vi "barcodeR092B.vi"(8 "主码":string, 10 "固定码":cluster{"start row":i32, "start column":i32}={"start row"=2, "start column"=1}) -> (2 "R92A二维码":string)   [LabVIEW 2020]
uses:
  Sources/Global_Variable/Global.vi
panel:
  out "结果字符串":string
  out "校验码":string="4"
  out "校验码数组":string[](array[string])=["0", "1", "2", "3", "4", "5", "6", "7", "8", "9", "A", "B", "C", "D", "E", "F", "G", "H", "J", "K", "L", "M", "N", "P", "R", "S", "T", "U", "V", "W", "X", "Y", "Z"]
  out "月份字码对照月校验数组":string[](array[string])=["", "", "", "", "", "", "", "", "", "", "01", "02", "03", "04", "05", "06", "07", "08", "09", "10", "11", "12"]
  out "批次流水号码":string
  out "年月日":string
  out "年月日时分码":string
  out "日期/时间字符串":string
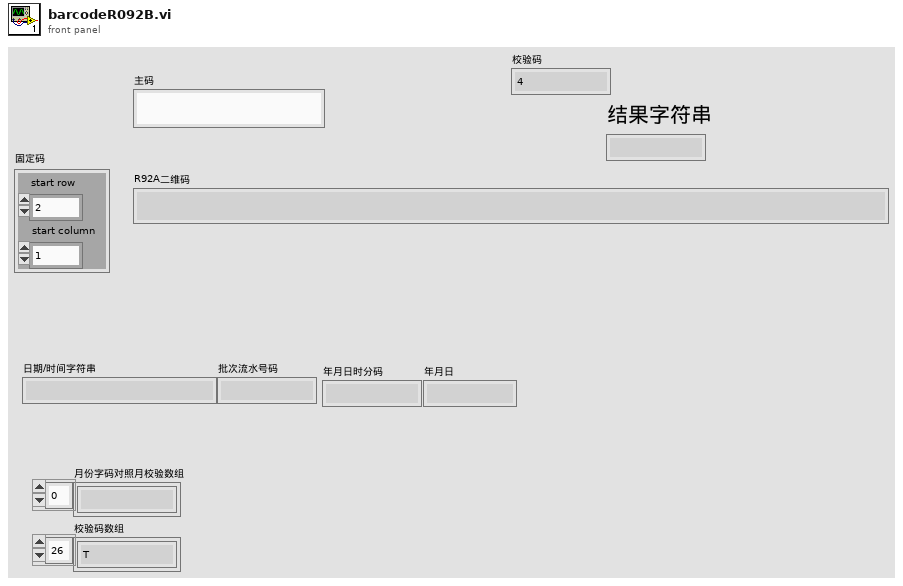
[diagram p1: front panel]
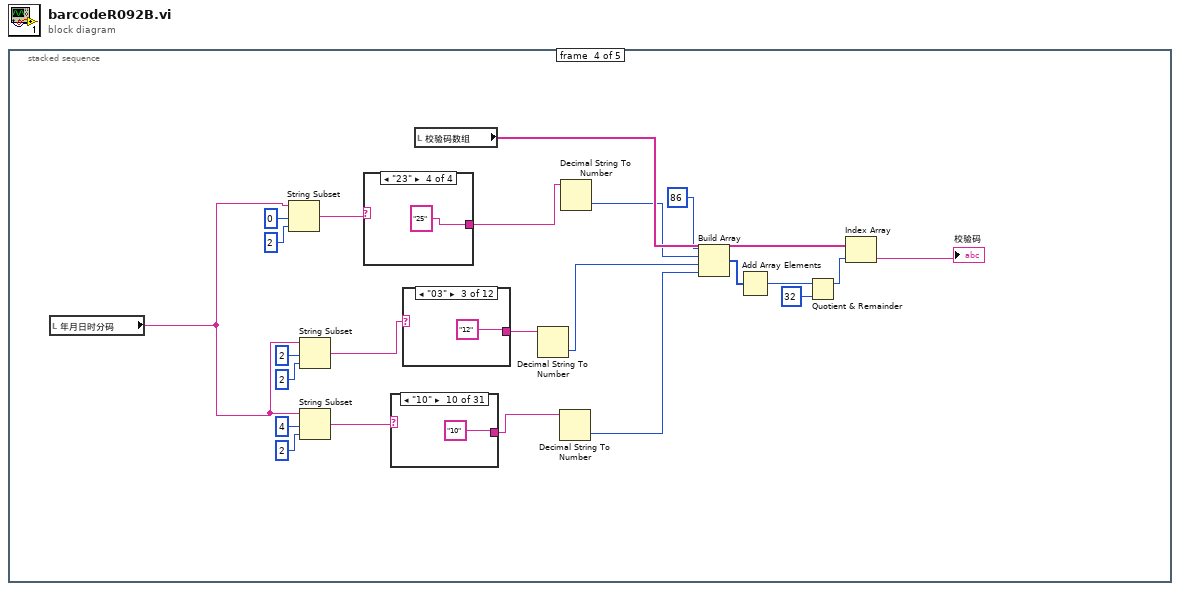
[diagram p0: block diagram]
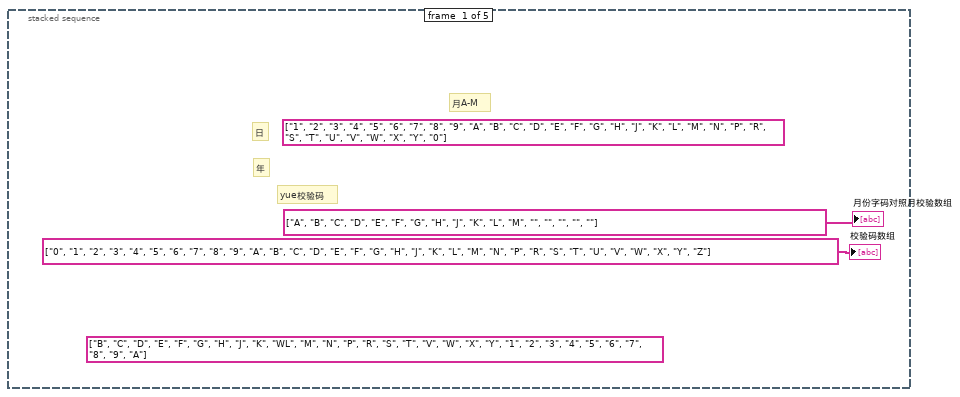
[diagram p2: hidden frame]
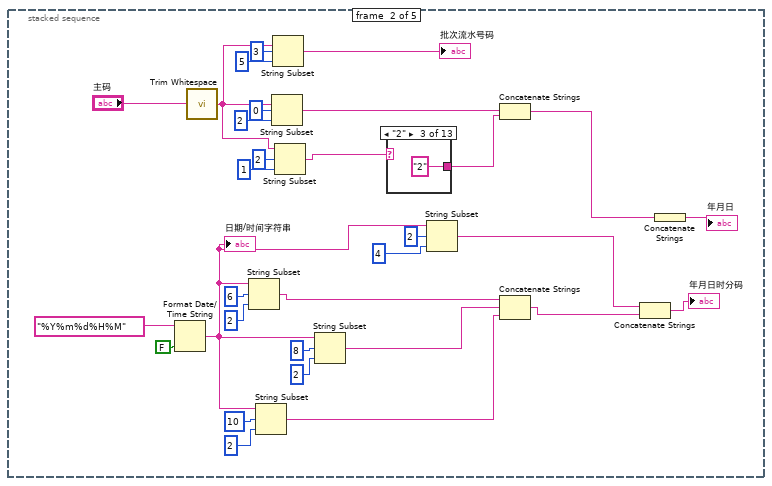
[diagram p3: hidden frame]
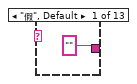
[diagram p4: hidden frame]
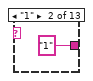
[diagram p5: hidden frame]
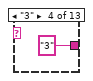
[diagram p6: hidden frame]
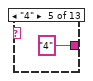
[diagram p7: hidden frame]
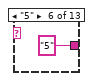
[diagram p8: hidden frame]
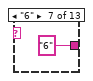
[diagram p9: hidden frame]
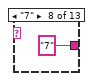
[diagram p10: hidden frame]
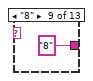
[diagram p11: hidden frame]
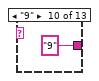
[diagram p12: hidden frame]
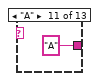
[diagram p13: hidden frame]
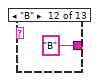
[diagram p14: hidden frame]
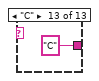
[diagram p15: hidden frame]
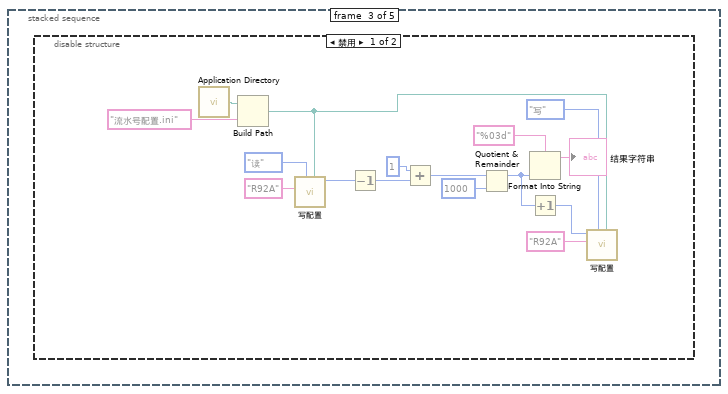
[diagram p16: hidden frame]
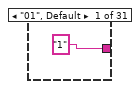
[diagram p18: hidden frame]
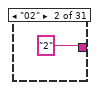
[diagram p19: hidden frame]
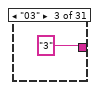
[diagram p20: hidden frame]
diagram:
  n1 = stacked-sequence {
    frame #0 {
      (unwired) string[] ["B", "C", "D", "E", "F", "G", "H", "J", "K", "WL", "M", "N", "P", "R", "S", "T", "V", "W", "X", "Y", "1", "2", "3", "4", "5", "6", "7", "8", "9", "A"]
      (unwired) string[] ["1", "2", "3", "4", "5", "6", "7", "8", "9", "A", "B", "C", "D", "E", "F", "G", "H", "J", "K", "L", "M", "N", "P", "R", "S", "T", "U", "V", "W", "X", "Y", "0"]
      # "月A-M"
      # "yue校验码"
      # "日"
      # "年"
      "月份字码对照月校验数组" <- string[] ["A", "B", "C", "D", "E", "F", "G", "H", "J", "K", "L", "M", "", "", "", "", ""]
      "校验码数组" <- string[] ["0", "1", "2", "3", "4", "5", "6", "7", "8", "9", "A", "B", "C", "D", "E", "F", "G", "H", "J", "K", "L", "M", "N", "P", "R", "S", "T", "U", "V", "W", "X", "Y", "Z"]
    }
    frame #1 {
      n2 = Format Date/Time String(time format string (%c)="%Y%m%d%H%M" ("时间格式字符串(%c)"), UTC format=FALSE ("UTC格式")) -> (date/time string=w7:string)  [unwired: 1 in]
      "日期/时间字符串" <- w7
      n3 = call <vilib>:"Trim Whitespace.vi"("string"="主码") -> ("trimmed string"=w11:string)  [unwired: 1 in]
      n4 = String Subset(string=w7, offset (0)=6 ("偏移量(0)"), length (rest)=2 ("长度（剩余）")) -> (substring=w14:string)
      n5 = String Subset(string=w7, offset (0)=10 ("偏移量(0)"), length (rest)=2 ("长度（剩余）")) -> (substring=w3:string)
      n6 = String Subset(string=w11, offset (0)=0 ("偏移量(0)"), length (rest)=2 ("长度（剩余）")) -> (substring=w20:string)
      n7 = String Subset(string=w11, offset (0)=3 ("偏移量(0)"), length (rest)=5 ("长度（剩余）")) -> (substring=→"批次流水号码":string)
      n8 = String Subset(string=w11, offset (0)=2 ("偏移量(0)"), length (rest)=1 ("长度（剩余）")) -> (substring=w21:string)
      n9 = String Subset(string=w7, offset (0)=8 ("偏移量(0)"), length (rest)=2 ("长度（剩余）")) -> (substring=w9:string)
      n10 = case shown="\"2\"" w21 {
        tunnel: ["" "1" "2" "3" "4" "5" "6" "7" "8" "9" "A" "B" "C"] -> w19
        frame "假", Default {
        }
        frame "1" {
        }
        frame "2" {
        }
        frame "3" {
        }
        frame "4" {
        }
        frame "5" {
        }
        frame "6" {
        }
        frame "7" {
        }
        frame "8" {
        }
        frame "9" {
        }
        frame "A" {
        }
        frame "B" {
        }
        frame "C" {
        }
      }
      n11 = String Subset(string=w7, offset (0)=2 ("偏移量(0)"), length (rest)=4 ("偏移量(0)")) -> (substring=w5:string)
      n12 = Concatenate Strings(w20, w19) -> (w8:string)
      n13 = Concatenate Strings(w14, w9, w3) -> (w18:string)
      n14 = Concatenate Strings(w5, w18) -> (→"年月日时分码":string)
      n15 = Concatenate Strings(w8) -> (→"年月日":string)
    }
    frame #2 {
      n16 = disable-structure shown="禁用" {
        frame Disabled {
          n17 = call <vilib>:"Application Directory.vi"() -> ("Application Directory"=w61:path)
          n18 = Build Path(base path=w61, name or relative path="流水号配置.ini" ("名称或相对路径")) -> (appended path=w60:path)
          n19 = call "写配置.vi"("配置文件路径"=w60, "枚举"=enum16{"写", "读"}."读", "section"="R92A") -> ("读取值"=w59:u32)  [unwired: 8 in]
          n20 = Decrement(x=w59) -> (x-1=w58:u32)
          n21 = Add(x=u32 1, y=w58) -> (x+y=w62:u32)
          n22 = Quotient & Remainder(x=w62, y=u32 1000) -> (x-y*floor(x/y)=w57:u32)  [unwired: 1 out]
          n23 = Format Into String(format string="%03d" ("格式字符串"), w57) -> (resulting string=→"结果字符串":string)  [unwired: 2 in, 1 out]
          n24 = Increment(x=w57) -> (x+1=w56:u32)
          n25 = call "写配置.vi"("配置文件路径"=w60, "枚举"=enum16{"写", "读"}."写", "section"="R92A", "写入值"=w56) -> ()  [unwired: 7 in, 1 out]
        }
        frame Enabled {
        }
      }
    }
    frame #3 {
      n26 = local read "年月日时分码"() -> (w71:string)
      n27 = String Subset(string=w71, offset (0)=0 ("偏移量(0)"), length (rest)=2 ("长度（剩余）")) -> (substring=w70:string)
      n28 = String Subset(string=w71, offset (0)=2 ("偏移量(0)"), length (rest)=2 ("长度（剩余）")) -> (substring=w67:string)
      n29 = String Subset(string=w71, offset (0)=4 ("偏移量(0)"), length (rest)=2 ("长度（剩余）")) -> (substring=w65:string)
      n30 = case shown="\"23\"" w70 {
        tunnel: ["21" "22" "23" "25"] -> w69
        frame "20", Default {
        }
        frame "21" {
        }
        frame "22" {
        }
        frame "23" {
        }
      }
      n31 = case shown="\"10\"" w65 {
        tunnel: ["1" "2" "3" "4" "5" "6" "7" "8" "9" "10" "11" "12" "13" "14" "15" "16" "17" "19" "20" "21" "22" "23" "25" "27" "28" "29" "30" "31" "32" "33" "34"] -> w64
        frame "01", Default {
        }
        frame "02" {
        }
        frame "03" {
        }
        frame "04" {
        }
        frame "05" {
        }
        frame "06" {
        }
        frame "07" {
        }
        frame "08" {
        }
        frame "09" {
        }
        frame "10" {
        }
        frame "11" {
        }
        frame "12" {
        }
        frame "13" {
        }
        frame "14" {
        }
        frame "15" {
        }
        frame "16" {
        }
        frame "17" {
        }
        frame "18" {
        }
        frame "19" {
        }
        frame "20" {
        }
        frame "21" {
        }
        frame "22" {
        }
        frame "23" {
        }
        frame "24" {
        }
        frame "25" {
        }
        frame "26" {
        }
        frame "27" {
        }
        frame "28" {
        }
        frame "29" {
        }
        frame "30" {
        }
        frame "31" {
        }
      }
      n32 = case shown="\"03\"" w67 {
        tunnel: ["10" "11" "12" "13" "14" "15" "16" "17" "19" "19" "21" "22"] -> w66
        frame "01", Default {
        }
        frame "02" {
        }
        frame "03" {
        }
        frame "04" {
        }
        frame "05" {
        }
        frame "06" {
        }
        frame "07" {
        }
        frame "08" {
        }
        frame "09" {
        }
        frame "10" {
        }
        frame "11" {
        }
        frame "12" {
        }
      }
      n33 = local read "校验码数组"() -> (w84:string[])
      n34 = Decimal String To Number(string=w66) -> (number=w72:i32)  [unwired: 2 in, 1 out]
      n35 = Decimal String To Number(string=w64) -> (number=w83:i32)  [unwired: 2 in, 1 out]
      n36 = Decimal String To Number(string=w69) -> (number=w82:i32)  [unwired: 2 in, 1 out]
      n37 = Build Array(86 ("元素"), w82, w72, w83) -> (w85:i32[])
      n38 = Add Array Elements(numeric array=w85) -> (sum=w81:i32)
      n39 = Quotient & Remainder(x=w81, y=32) -> (x-y*floor(x/y)=w63:i32)  [unwired: 1 out]
      n40 = Index Array(array=w84, index=w63) -> (element=→"校验码":string)
    }
    frame #4 {
      w136 = "*" ("字符串")
      # "返工码"
      # "生产日期+批次号"
      # "固定码"
      n41 = disable-structure shown="禁用" {
        frame Disabled {
          n42 = call "ReadexcelR092B.vi"("start (0, 0)"=cluster{"start row":i32, "start column":i32} {"start row"=7, "start column"=3}) -> ()  [unwired: 10 in, 1 out]
          n43 = call "ReadexcelR092B.vi"("start (0, 0)"=cluster{"start row":i32, "start column":i32} {"start row"=7, "start column"=4}) -> ()  [unwired: 10 in, 1 out]
          n44 = call "ReadexcelR092B.vi"("start (0, 0)"=cluster{"start row":i32, "start column":i32} {"start row"=7, "start column"=1}) -> ()  [unwired: 10 in, 1 out]
        }
        frame Enabled {
        }
      }
      n45 = global read "Global.vi" "追溯代码"() -> (w135:string)
      n46 = global read "Global.vi" "返工码"() -> (w133:string)
      n47 = global read "Global.vi" "白/夜班"() -> (w134:string)
      n48 = local read "年月日时分码"() -> (w142:string)
      n49 = local read "批次流水号码"() -> (w140:string)
      n50 = local read "年月日"() -> (w141:string)
      n51 = local read "校验码"() -> (w139:string)
      n52 = Concatenate Strings(w142, "*" ("字符串"), w134, w141, w140) -> (w143:string)
      n53 = Concatenate Strings(w135, w143, "*安徽芜湖*1**" ("字符串"), w139, w136, w133, w136) -> (→"R92A二维码":string)
    }
  }
